vi "CreateControls.vi"(8 "error in":errorcluster, 11 "PythonConverter_GUI in":refnum<class "PythonConverter_GUI.lvclass">) -> (0 "error out":errorcluster, 3 "PythonConverter_GUI out":refnum<class "PythonConverter_GUI.lvclass">)   [LabVIEW 2014, in "PythonConverter_GUI.lvclass"]
uses:
  PythonConverter_GUI.lvclass
  PythonConverter_GUI.lvclass/PythonConverter_GUI.ctl
  VI Interpreter/Classes/Control/ImageTypes.ctl
  VI Interpreter/Classes/Control/Control.lvclass
  VI Interpreter/Classes/VI Interpreter/VI Interpreter.lvclass
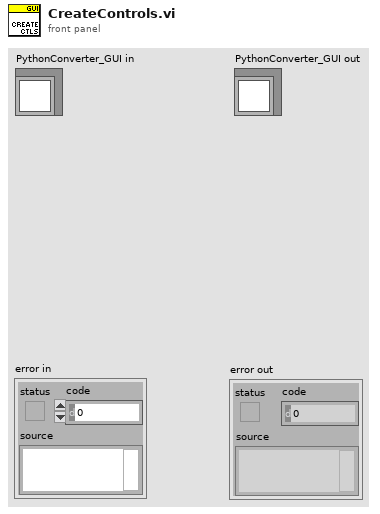
[diagram p1: front panel]
types:
  T1 = typedef "PythonConverter_GUI.lvclass/PythonModuleTD.ctl" = cluster{"Python module":string, "Python module  name":string}
  T2 = typedef "ImageTypes.ctl" = enum16{"PNG", "JPEG", "BMP"}
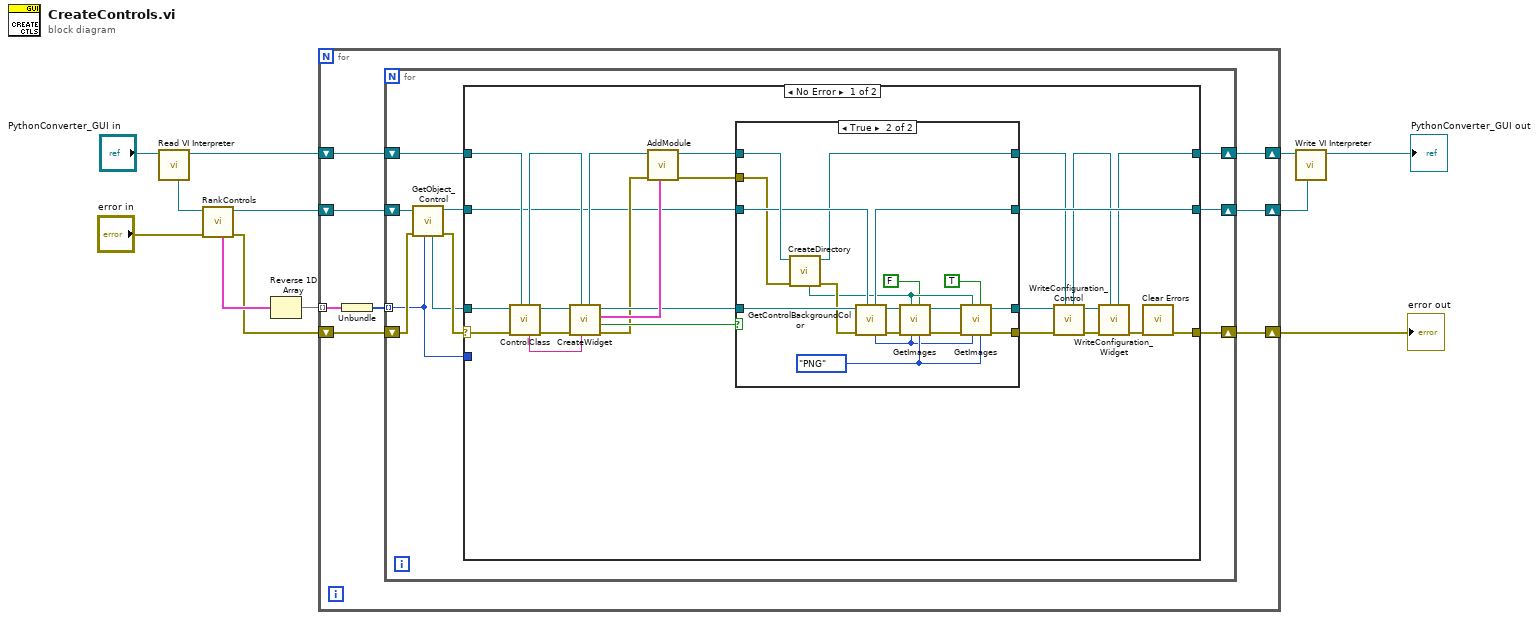
[diagram p0: block diagram]
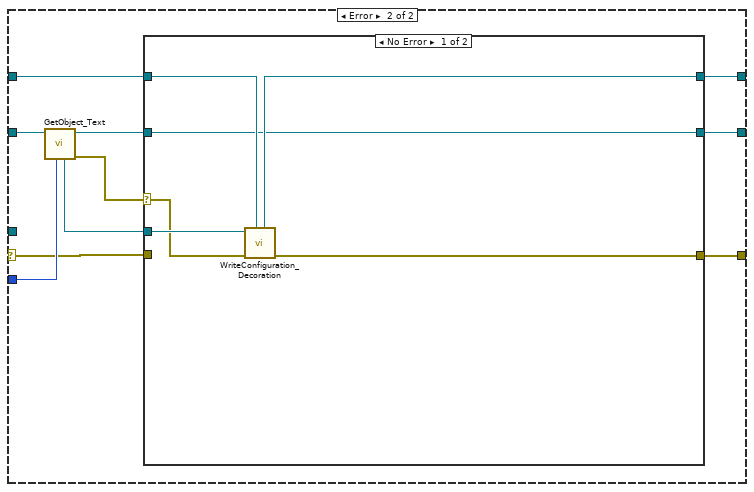
[diagram p3: hidden frame]
diagram:
  n1 = call "Read VI Interpreter.vi"("PythonConverter_GUI in"="PythonConverter_GUI in") -> ("PythonConverter_GUI out"=w6:refnum<class "PythonConverter_GUI.lvclass">, "VI Interpreter"=w5:refnum<class "VI Interpreter.lvclass">)  [unwired: 7 in]
  n2 = call "RankControls.vi"("error in"="error in", "VI Interpreter in"=w5) -> ("error out"=w10:errorcluster, "VI Interpreter out"=w8:refnum<class "VI Interpreter.lvclass">, "Rank"=w11:cluster{"nodes":i32[]}[])  [unwired: 5 in]
  n3 = Reverse 1D Array(array=w11) -> (reversed array=w1:cluster{"nodes":i32[]}[])
  n4 = for {
    tunnel: w1 -> [w18] mode=indexing
    shift-right: [w15] -> w2
    shift-left: w8 -> [w16]
    shift-right: [w19] -> w9
    shift-left: w10 -> [w20]
    shift-right: [w13] -> w4
    shift-left: w6 -> [w14]
    n5 = Unbundle(w18) -> ("nodes"=w17:i32[])
    n6 = for {
      shift-right: [w30] -> w19
      shift-left: w20 -> [w28]
      tunnel: w17 -> [w21] mode=indexing
      shift-right: [w24] -> w15
      shift-left: w16 -> [w29]
      shift-right: [w22] -> w13
      shift-left: w14 -> [w23]
      n7 = call "GetObject_Control.vi"("UID"=w21, "error in"=w28, "VI Interpreter in"=w29) -> ("error out"=w27:errorcluster, "VI Interpreter out"=w25:refnum<class "VI Interpreter.lvclass">, "control"=w26:refnum<class "Control.lvclass">)  [unwired: 3 in, 1 out]
      n8 = case shown="No Error" w27 {
        selector: w27 -> [w36 w83]
        tunnel: [w55 w82] -> w30
        tunnel: w26 -> [w37 _]
        tunnel: w25 -> [w31 w87]
        tunnel: [w48 w80] -> w24
        tunnel: w23 -> [w38 w79]
        tunnel: [w39 w78] -> w22
        tunnel: w21 -> [_ w86]
        frame No Error {
          n9 = call "ControlClass.vi"("PythonConverter_GUI in"=w38, "error in"=w36, "Control in"=w37) -> ("error out"=w33:errorcluster, "Control out"=w34:refnum<class "Control.lvclass">, "control name"=w32:string, "PythonConverter_GUI out"=w35:refnum<class "PythonConverter_GUI.lvclass">)  [unwired: 5 in]
          n10 = call "CreateWidget.vi"("control name"=w32, "PythonConverter_GUI in"=w35, "error in"=w33, "Control in"=w34) -> ("error out"=w50:errorcluster, "get image"=w52:bool, "module"=w54:T1, "Control out"=w51:refnum<class "Control.lvclass">, "PythonConverter_GUI out"=w53:refnum<class "PythonConverter_GUI.lvclass">)  [unwired: 2 in, 1 out]
          n11 = call "AddModule.vi"("module"=w54, "error in"=w50, "PythonConverter_GUI in"=w53) -> ("error out"=w47:errorcluster, "PythonConverter_GUI out"=w49:refnum<class "PythonConverter_GUI.lvclass">)  [unwired: 5 in]
          n12 = case shown="True" w52 {
            tunnel: w51 -> [w56 w70]
            tunnel: w49 -> [w59 w77]
            tunnel: w31 -> [w58 w76]
            tunnel: [w58 w75] -> w48
            tunnel: [w59 w74] -> w44
            tunnel: [w57 w65] -> w46
            tunnel: w47 -> [w57 w73]
            tunnel: [w56 w66] -> w45
            frame False {
            }
            frame True {
              w64 = ImageTypes."PNG" ("File type")
              n13 = call "CreateDirectory.vi"("error in"=w73, "PythonConverter_GUI in"=w77) -> ("error out"=w69:errorcluster, "PythonConverter_GUI out"=w74:refnum<class "PythonConverter_GUI.lvclass">, "Path"=w62:path)  [unwired: 5 in]
              n14 = call "GetControlBackgroundColor.vi"("VI Interpreter in"=w76, "error in"=w69, "Control in"=w70) -> ("error out"=w72:errorcluster, "Control out"=w71:refnum<class "Control.lvclass">, "BG color"=w63:u32, "VI Interpreter out"=w75:refnum<class "VI Interpreter.lvclass">)  [unwired: 5 in]
              n15 = call-dynamic "GetImages.vi"("File type"=w64, "Disabled"=FALSE, "Background Color"=w63, "image directory"=w62, "error in"=w72, "Control in"=w71) -> ("error out"=w68:errorcluster, "Control out"=w67:refnum<class "Control.lvclass">)  [unwired: 4 in]
              n16 = call-dynamic "GetImages.vi"("File type"=w64, "Disabled"=TRUE, "Background Color"=w63, "image directory"=w62, "error in"=w68, "Control in"=w67) -> ("error out"=w65:errorcluster, "Control out"=w66:refnum<class "Control.lvclass">)  [unwired: 4 in]
            }
          }
          n17 = call "WriteConfiguration_Control.vi"("PythonConverter_GUI in"=w44, "error in"=w46, "Control in"=w45) -> ("error out"=w43:errorcluster, "Control out"=w42:refnum<class "Control.lvclass">, "PythonConverter_GUI out"=w40:refnum<class "PythonConverter_GUI.lvclass">)  [unwired: 6 in]
          n18 = call "WriteConfiguration_Widget.vi"("PythonConverter_GUI in"=w40, "error in"=w43, "Control in"=w42) -> ("error out"=w41:errorcluster, "PythonConverter_GUI out"=w39:refnum<class "PythonConverter_GUI.lvclass">)  [unwired: 6 in, 1 out]
          n19 = call <vilib>:"Clear Errors.vi"("error in (no error)"=w41) -> ("error out"=w55:errorcluster)  [unwired: 5 in, 1 out]
        }
        frame Error {
          n20 = call "GetObject_Text.vi"("UID"=w86, "VI Interpreter in"=w87) -> ("error out"=w84:errorcluster, "VI Interpreter out"=w85:refnum<class "VI Interpreter.lvclass">, "Text"=w81:refnum<class "Text.lvclass">)  [unwired: 4 in, 1 out]
          n21 = case shown="No Error" w84 {
            selector: w84 -> [w89 _]
            tunnel: w85 -> [w88 w95]
            tunnel: w83 -> [_ _]
            tunnel: [w91 _] -> w82
            tunnel: w81 -> [w90 _]
            tunnel: [w88 w95] -> w80
            tunnel: w79 -> [w93 w94]
            tunnel: [w92 w94] -> w78
            frame No Error {
              n22 = call "WriteConfiguration_Decoration.vi"("PythonConverter_GUI in"=w93, "error in"=w89, "Decoration in"=w90) -> ("error out"=w91:errorcluster, "PythonConverter_GUI out"=w92:refnum<class "PythonConverter_GUI.lvclass">)  [unwired: 6 in, 1 out]
            }
            frame Error {
            }
          }
        }
      }
    }
  }
  "error out" <- w9
  n23 = call "Write VI Interpreter.vi"("VI Interpreter"=w2, "PythonConverter_GUI in"=w4) -> ("PythonConverter_GUI out"=→"PythonConverter_GUI out":refnum<class "PythonConverter_GUI.lvclass">)  [unwired: 7 in]
